vi "Main_Backup00.vi"() -> ()   [LabVIEW 2024]
uses:
  ConfigPIMax3Two/x64/Release/ConfigPIMax3Two.dll
  PIMax3Test01/x64/Debug/PIMax3Test01.dll
panel:
  out "Intensity Graph 2":u16[][](graph)
  out "image":i32[](array[numeric])
  out "Uninit Message":string
  out "close":string
  out "model":string
  out "open":string
  out "Init Message":string
  out "Uninit Code":i32
  out "Init Code":i32
  out "c 2":i32
  out "c":i32
  in  "b":i32=3
  in  "a":i32=5
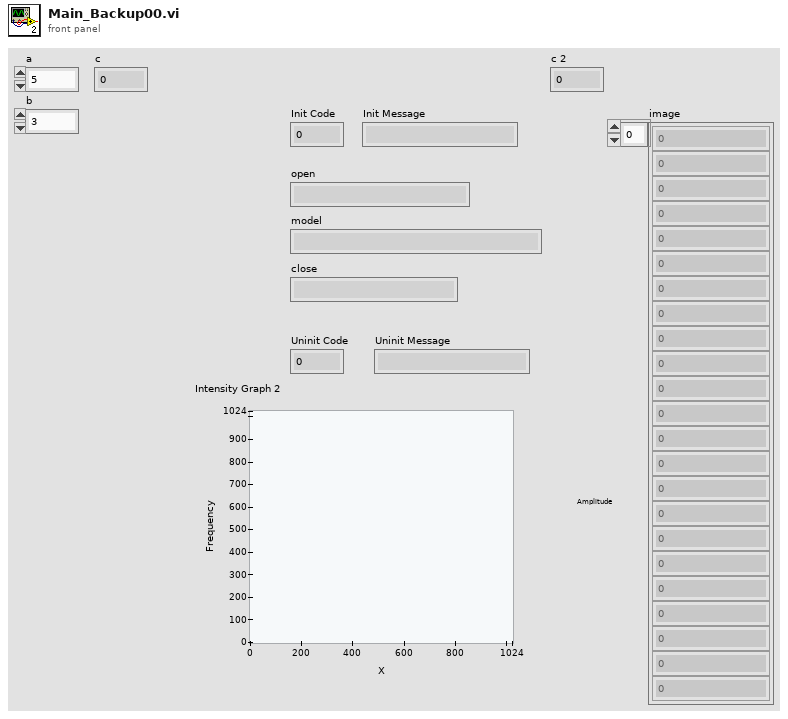
[diagram p1: front panel]
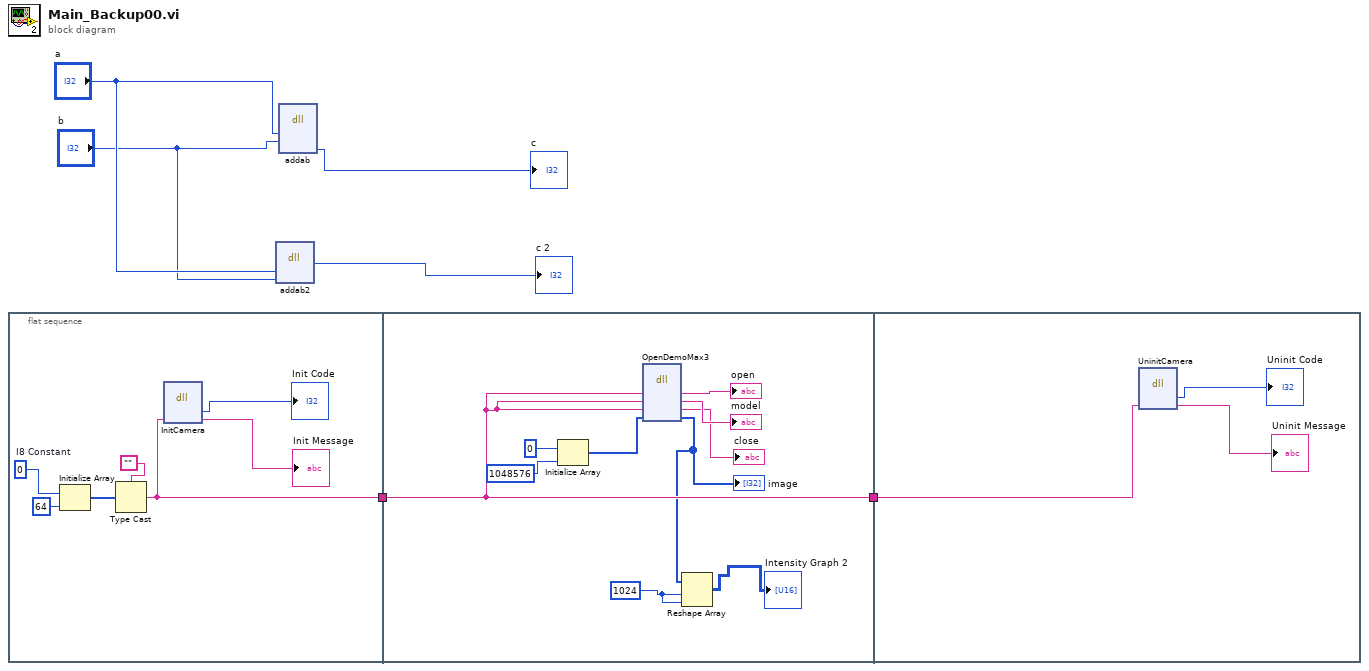
[diagram p0: block diagram]
diagram:
  n1 = flat-sequence {
    tunnel: [w7] -> w2
    tunnel: w2 -> [w20]
    tunnel: [w20] -> w1
    tunnel: w1 -> [w25]
    frame #0 {
      w12 = i8 0  # I8 Constant
      n2 = Initialize Array(w12, 64 ("dimension size")) -> (w11:i8[])
      n3 = Type Cast(type="", x=w11) -> (*(type *) &x=w7:string)
      n4 = dll-call lib="C:/Users/amir0/source/repos/PIMax3Test01/x64/Debug/PIMax3Test01.dll" fn="InitCamera"("Init Message"=w7) -> ("Init Code"=→"Init Code":i32, "Init Message"=→"Init Message":string)  [unwired: 5 in, 2 out]
    }
    frame #1 {
      w15 = 1024 ("dimension size")
      n5 = Initialize Array(u16 0, 1048576 ("dimension size")) -> (w18:u16[])
      n6 = dll-call lib="C:/Users/amir0/source/repos/PIMax3Test01/x64/Debug/PIMax3Test01.dll" fn="OpenDemoMax3"("open"=w20, "model"=w20, "close"=w20, "image"=w18) -> ("open"=→"open":string, "model"=→"model":string, "close"=→"close":string, "image"=w16:u16[])  [unwired: 4 in, 2 out]
      "image" <- w16
      n7 = Reshape Array(w16, w15, w15) -> (→"Intensity Graph 2":u16[][])
    }
    frame #2 {
      n8 = dll-call lib="C:/Users/amir0/source/repos/PIMax3Test01/x64/Debug/PIMax3Test01.dll" fn="UninitCamera"("Uninit Message"=w25) -> ("Uninit Code"=→"Uninit Code":i32, "Uninit Message"=→"Uninit Message":string)  [unwired: 5 in, 2 out]
    }
  }
  n9 = dll-call lib="C:/Users/amir0/source/repos/ConfigPIMax3Two/x64/Release/ConfigPIMax3Two.dll" fn="addab2"("a"="a", "b"="b") -> ("return type"=→"c 2":i32)  [unwired: 5 in, 2 out]
  n10 = dll-call lib="C:/Users/amir0/source/repos/ConfigPIMax3Two/x64/Release/ConfigPIMax3Two.dll" fn="addab"("a"="a", "b"="b") -> ("c"=→"c":i32)  [unwired: 7 in, 2 out]
